vi "Get All Compiled Messages and Subaddresses.vi"(8 "error in":errorcluster, 11 "custom device ref":T2 format="%.0x") -> (0 "error out":errorcluster, 2 "all messages and subaddresses":T1[](array[typedef]) {"Timestamp Channel Handle" format="%.0x"; "Message Section Handle" format="%.0x"; "Parameter Channel Handles" format="%.0x"}, 3 "custom device ref out":T2 format="%.0x")   [LabVIEW 2020, in "AIM MIL-STD-1553 Engine.lvlib" / "Implementation.lvlib" / "Execution Unit.lvclass"]
uses:
  Execution Unit.lvclass
  <vilib>/NI VeriStand/Custom Device API/Custom Device Item Ref.ctl
  Custom Device/Compiled Message.ctl
  Shared/Direction.ctl
  Shared/Parameter Definition.ctl
  <vilib>/NI VeriStand/Custom Device API/Custom Device API.lvlib
  Scripting/AIM MIL-STD-1553 Scripting.lvlib
  Custom Device/Custom Device.lvlib
  <vilib>/NI VeriStand/Custom Device Tools/Custom Device Utility Library/Custom Device Utility Library.lvlib
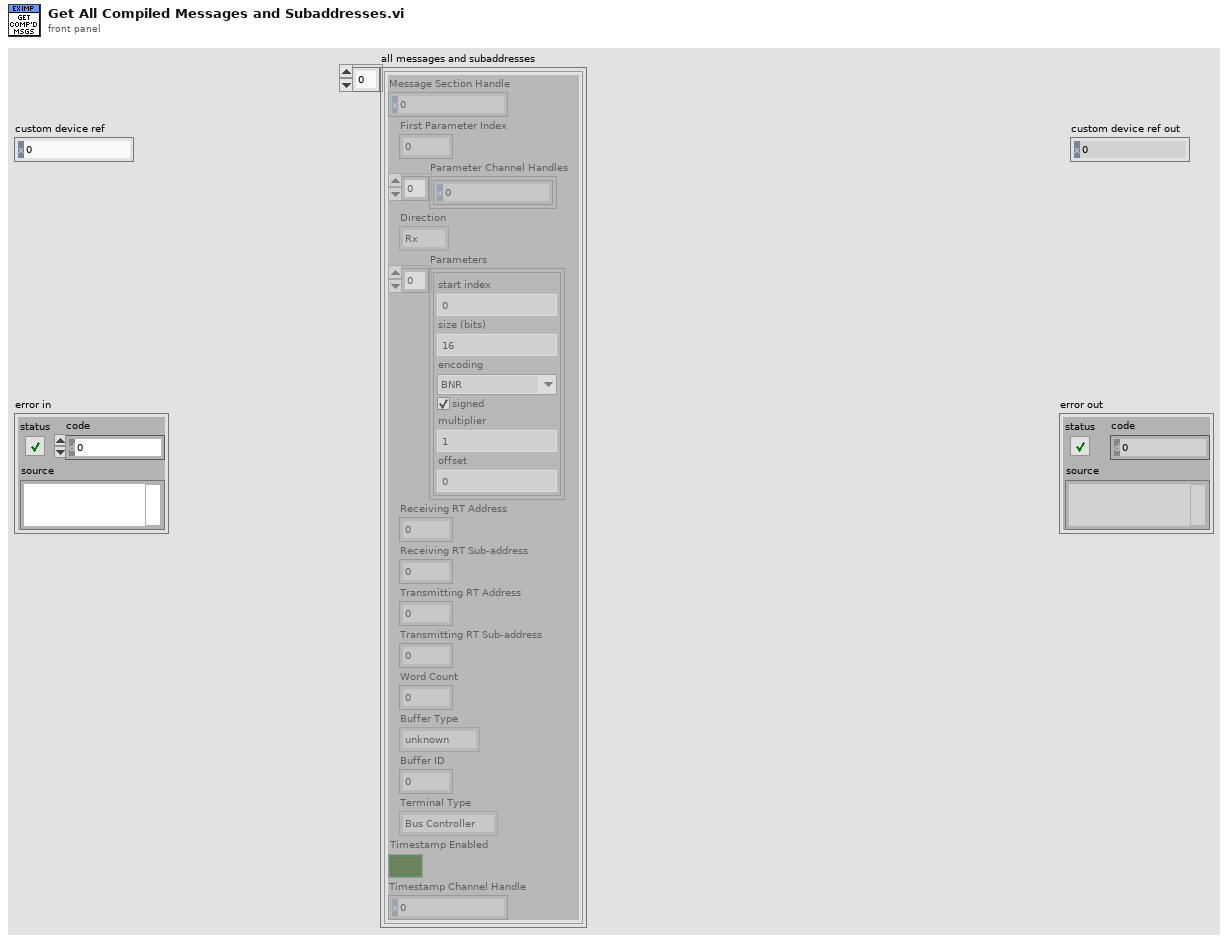
[diagram p1: front panel]
types:
  T1 = typedef "AIM MIL-STD-1553 Engine.lvlib/Custom Device.lvlib/Compiled Message.ctl" = cluster{"Message Section Handle":T2, "First Parameter Index":i32, "Parameter Channel Handles":T2[], "Direction":T3, "Parameters":T4[], "Receiving RT Address":u8, "Receiving RT Sub-address":u8, "Transmitting RT Address":u8, "Transmitting RT Sub-address":u8, "Word Count":u8, "Buffer Type":enum16{"unknown", "BC Message Buffer", "RT Message Buffer"}, "Buffer ID":u16, "Terminal Type":enum16{"Bus Controller", "Remote Terminal"}, "Timestamp Enabled":bool, "Timestamp Channel Handle":T2}
  T2 = typedef "Custom Device API.lvlib/Custom Device Item Ref.ctl" = u64
  T3 = typedef "Direction.ctl" = enum16{"Rx", "Tx"}
  T4 = typedef "Parameter Definition.ctl" = cluster{"start index":i32, "size (bits)":i32, "encoding":enum16{"BNR", "BCD", "Discrete"}, "signed":bool, "multiplier":dbl, "offset":dbl}
  T5 = typedef "Terminal Endpoint.ctl" = cluster{"terminal address":T6, "subaddress":T6}
  T6 = typedef "Address.ctl" = u16
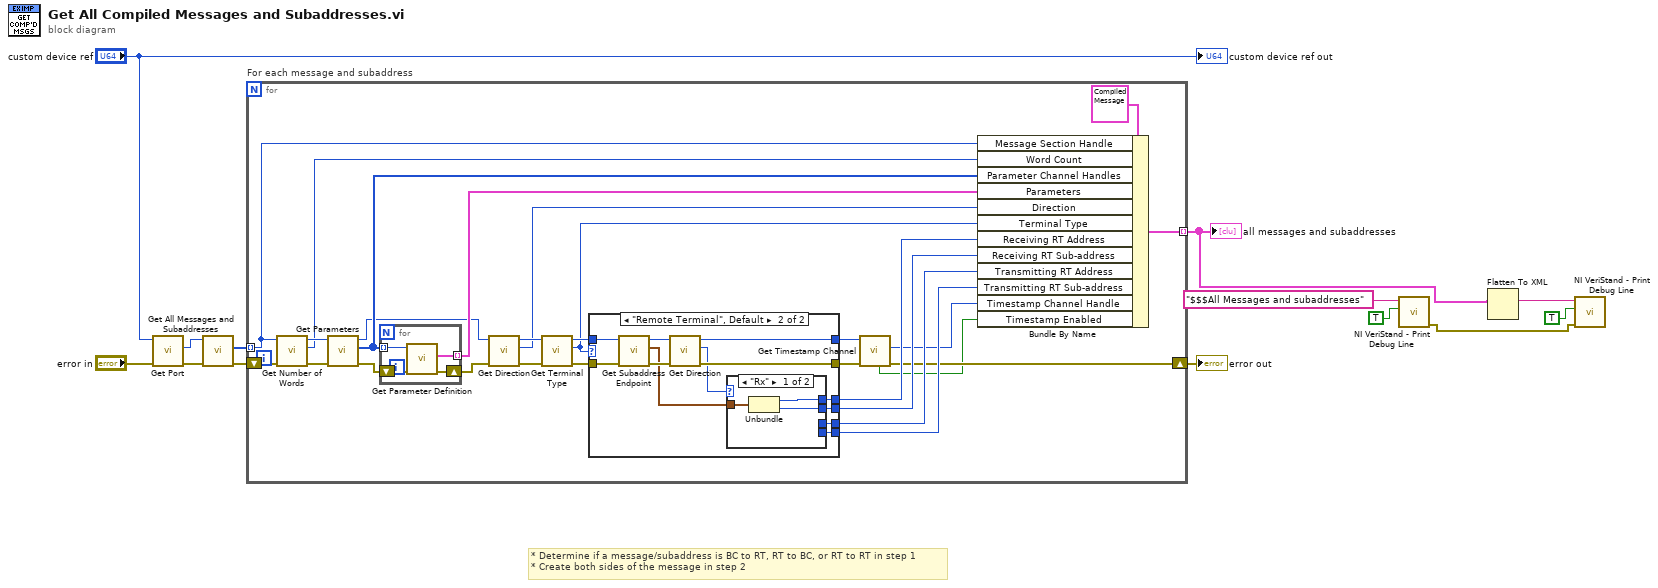
[diagram p0: block diagram]
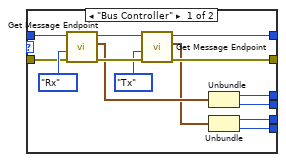
[diagram p2: hidden frame]
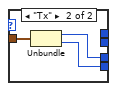
[diagram p3: hidden frame]
diagram:
  # "* Determine if a message/subaddress is BC to RT, RT to BC, or RT to RT in step 1\n* Create both sides of the message in step 2"
  n1 = call "Get Port.vi"("error in"="error in", "custom device ref"="custom device ref") -> ("error out"=w9:errorcluster, "port"=w8:T2)  [unwired: 6 in, 2 out]
  n2 = call "Get All Messages and Subaddresses.vi"("error in"=w9, "port"=w8) -> ("error out"=w13:errorcluster, "messages and subaddresses"=w12:T2[])  [unwired: 7 in, 1 out]
  n3 = for "For each message and subaddress" {
    shift-right: [w22] -> w7
    shift-left: w13 -> [w16]
    tunnel: w12 -> [w18] mode=indexing
    tunnel: [w14] -> w1 mode=indexing
    n4 = call "Get Number of Words.vi"("error in"=w16, "message or subaddress"=w18) -> ("error out"=w27:errorcluster, "number of words"=w25:u16, "message or subaddress out"=w26:T2)  [unwired: 7 in]
    n5 = call "Get Parameters.vi"("error in"=w27, "message or subaddress"=w26) -> ("error out"=w39:errorcluster, "parameters"=w38:T2[], "message or subaddress out"=w15:T2)  [unwired: 7 in]
    n6 = for {
      shift-right: [w76] -> w36
      shift-left: w39 -> [w75]
      tunnel: w38 -> [w74] mode=indexing
      tunnel: [w73] -> w37 mode=indexing
      n7 = call "Get Parameter Definition.vi"("error in"=w75, "parameter"=w74) -> ("error out"=w76:errorcluster, "parameter definition"=w73:T4)  [unwired: 7 in, 1 out]
    }
    n8 = call "Get Direction.vi"("error in"=w36, "message or subaddress"=w15) -> ("error out"=w33:errorcluster, "direction"=w17:T3, "message or subaddress out"=w32:T2)  [unwired: 6 in, 1 out]
    n9 = call "Get Terminal Type.vi"("error in"=w33, "message or subaddress"=w32) -> ("error out"=w35:errorcluster, "terminal type"=w24:enum16{"Bus Controller", "Remote Terminal"}, "message or subaddress out"=w34:T2)  [unwired: 7 in]
    n10 = case shown="\"Remote Terminal\", Default" w24 {
      tunnel: [w48 w64] -> w21
      tunnel: [w47 w63] -> w23
      tunnel: w34 -> [w54 w60]
      tunnel: w35 -> [w52 w59]
      tunnel: [w41 w58] -> w28
      tunnel: [w42 w57] -> w29
      tunnel: [w45 w56] -> w30
      tunnel: [w46 w55] -> w31
      frame "Bus Controller" {
        n11 = call "Get Message Endpoint.vi"("error in"=w52, "direction"=Direction."Rx", "message"=w54) -> ("error out"=w51:errorcluster, "remote terminal endpoint"=w44:T5, "message out"=w49:T2)  [unwired: 5 in, 1 out]
        n12 = call "Get Message Endpoint.vi"("error in"=w51, "direction"=Direction."Tx", "message"=w49) -> ("error out"=w47:errorcluster, "remote terminal endpoint"=w43:T5, "message out"=w48:T2)  [unwired: 5 in, 1 out]
        n13 = Unbundle(w44) -> ("terminal address"=w46:T6, "subaddress"=w45:T6)
        n14 = Unbundle(w43) -> ("terminal address"=w42:T6, "subaddress"=w41:T6)
      }
      frame "Remote Terminal", Default {
        n15 = call "Get Subaddress Endpoint.vi"("error in"=w59, "subaddress"=w60) -> ("error out"=w65:errorcluster, "remote terminal endpoint"=w61:T5, "subaddress out"=w66:T2)  [unwired: 7 in]
        n16 = call "Get Direction.vi"("error in"=w65, "message or subaddress"=w66) -> ("error out"=w63:errorcluster, "direction"=w62:T3, "message or subaddress out"=w64:T2)  [unwired: 6 in, 1 out]
        n17 = case shown="\"Rx\"" w62 {
          tunnel: w61 -> [w69 w72]
          tunnel: [w68 _] -> w55
          tunnel: [w67 _] -> w56
          tunnel: [_ w71] -> w57
          tunnel: [_ w70] -> w58
          frame "Rx" {
            n18 = Unbundle(w69) -> ("terminal address"=w68:T6, "subaddress"=w67:T6)
          }
          frame "Tx" {
            n19 = Unbundle(w72) -> ("terminal address"=w71:T6, "subaddress"=w70:T6)
          }
        }
      }
    }
    n20 = call "Get Timestamp Channel.vi"("error in"=w23, "message section"=w21) -> ("error out"=w22:errorcluster, "timestamp channel"=w19:T2, "found?"=w20:bool)  [unwired: 6 in, 1 out]
    n21 = Bundle By Name(cluster=T1 {"Message Section Handle"=18446744073709551615, "First Parameter Index"=0, "Parameter Channel Handles"=[], "Direction"=enum."Rx", "Parameters"=[], "Receiving RT Address"=0, "Receiving RT Sub-address"=0, "Transmitting RT Address"=0, "Transmitting RT Sub-address"=0, "Word Count"=0, "Buffer Type"=enum."unknown", "Buffer ID"=0, "Terminal Type"=enum."Bus Controller", "Timestamp Enabled"=FALSE, "Timestamp Channel Handle"=0}, "Message Section Handle"=w18, "Word Count"=w25, "Parameter Channel Handles"=w38, "Parameters"=w37, "Direction"=w17, "Terminal Type"=w24, "Receiving RT Address"=w31, "Receiving RT Sub-address"=w30, "Transmitting RT Address"=w29, "Transmitting RT Sub-address"=w28, "Timestamp Channel Handle"=w19, "Timestamp Enabled"=w20) -> (w14:T1)
  }
  "error out" <- w7
  "all messages and subaddresses" <- w1
  n22 = call <vilib>:"NI VeriStand - Print Debug Line.vi"("Add to log file? (F)"=TRUE, "Message"="$$$All Messages and subaddresses") -> ("error out"=w2:errorcluster)  [unwired: 9 in]
  n23 = Flatten To XML(6:w1) -> (2:w6:string)
  n24 = call <vilib>:"NI VeriStand - Print Debug Line.vi"("error in (no error)"=w2, "Add to log file? (F)"=TRUE, "Message"=w6) -> ()  [unwired: 8 in, 1 out]
  "custom device ref out" <- "custom device ref"
